vi "XY Graph Show-Hide Tool Panels.vi"(8 "Error In":errorcluster, 9 "Hide (F) /Show (T)":bool, 11 "XY Graph Ref":T1) -> (0 "Error Out":errorcluster, 1 "Tool Panels Shown?":bool)   [LabVIEW 2021, in "XY Graph Add-Ons.lvlib"]
uses:
  XY Graph Add-Ons.lvlib
  XY Graph Refnum.ctl
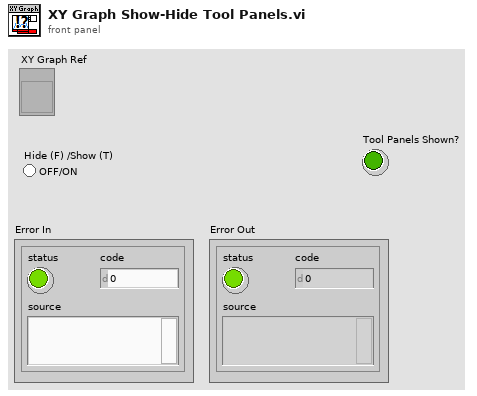
[diagram p1: front panel]
types:
  T1 = typedef "XY Graph Add-Ons.lvlib/XY Graph Refnum.ctl" = refnum<vi>
  T2 = typedef "XY Graph Add-Ons.lvlib/XY Graph Tool Panels Visibility.ctl" = cluster{"Scale Legend Vis":bool, "X-Scrollbar Vis":bool, "Cursor Panel Vis":bool, "Graph Palette Vis":bool}
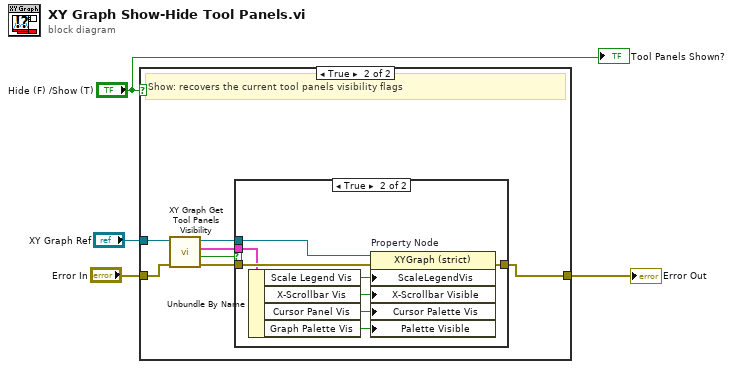
[diagram p0: block diagram]
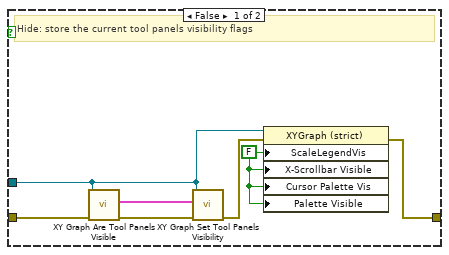
[diagram p2: hidden frame]
diagram:
  n1 = case shown="True" "Hide (F) /Show (T)" {
    tunnel: "XY Graph Ref" -> [w8 w17]
    tunnel: "Error In" -> [w11 w16]
    tunnel: [w5 w12] -> w2
    frame False {
      w6 = FALSE ("Scale Legend:Visible")
      # "Hide: store the current tool panels visibility flags"
      n2 = call "XY Graph Are Tool Panels Visible.vi"("Error In"=w11, "XY Graph Ref"=w8) -> ("Error Out"=w9:errorcluster, "Graph Tool Panels Visibility"=w10:T2)  [unwired: 6 in, 2 out]
      n3 = call "XY Graph Set Tool Panels Visibility.vi"("error in (no error)"=w9, "Graph Tool Panels Visibility"=w10, "XYGraph in"=w8) -> ("error out"=w7:errorcluster)  [unwired: 7 in, 1 out]
      n4 = property class="XYGraph (strict)"(reference=w8, error in=w7, "ScaleLegendVis"=w6, "X-Scrollbar Visible"=w6, "Cursor Palette Vis"=w6, "Palette Visible"=w6) -> (error out=w5:errorcluster)  [unwired: 1 out]
    }
    frame True {
      # "Show: recovers the current tool panels visibility flags"
      n5 = call "XY Graph Get Tool Panels Visibility.vi"("error in (no error)"=w16, "XYGraph in"=w17) -> ("error out"=w18:errorcluster, "Was Tag Found?"=w15:bool, "Graph Tool Panels Visibility"=w13:T2, "XYGraph out"=w14:T1)  [unwired: 6 in]
      n6 = case shown="True" w15 {
        tunnel: w13 -> [_ w24]
        tunnel: w18 -> [w19 w25]
        tunnel: w14 -> [_ w27]
        tunnel: [w19 w26] -> w12
        frame False {
        }
        frame True {
          n7 = Unbundle By Name(w24) -> ("Scale Legend Vis"=w23:bool, "X-Scrollbar Vis"=w22:bool, "Cursor Panel Vis"=w21:bool, "Graph Palette Vis"=w20:bool)
          n8 = property on="Property Node" class="XYGraph (strict)"(reference=w27, error in=w25, "ScaleLegendVis"=w23, "X-Scrollbar Visible"=w22, "Cursor Palette Vis"=w21, "Palette Visible"=w20) -> (error out=w26:errorcluster)  [unwired: 1 out]
        }
      }
    }
  }
  "Error Out" <- w2
  "Tool Panels Shown?" <- "Hide (F) /Show (T)"
